vi "Tri-Tri minimum separation.vi"(2 "Triangle 2":T1, 3 "Triangle 1":T1) -> (0 "Minimum separation distance":sgl, 1 "Minimum separation vector\nfrom triangle 2 to triange 1":sgl[](array[numeric]))   [LabVIEW 2014]
uses:
  Typedefs/Triangle.ctl
panel:
  # "PN 13/01/2015"
  # "Vertices"
  # "Edges"
  # "Unit normal"
  # "Edge unit normals"
  # "Vertices"
  # "Edges"
  # "Unit normal"
  # "Edge unit normals"
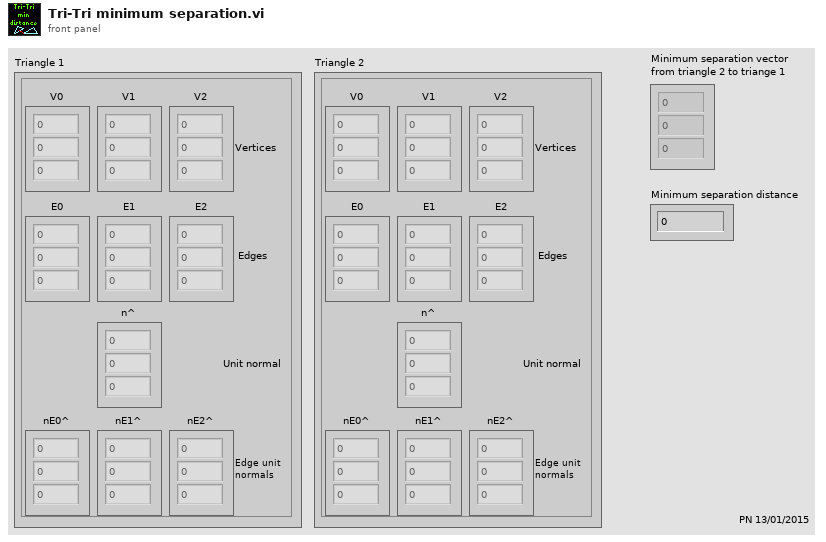
[diagram p1: front panel]
types:
  T1 = typedef "Triangle.ctl" = cluster{"V0":sgl[], "V1":sgl[], "V2":sgl[], "E0":sgl[], "E1":sgl[], "E2":sgl[], "n^":sgl[], "nE0^":sgl[], "nE1^":sgl[], "nE2^":sgl[]}
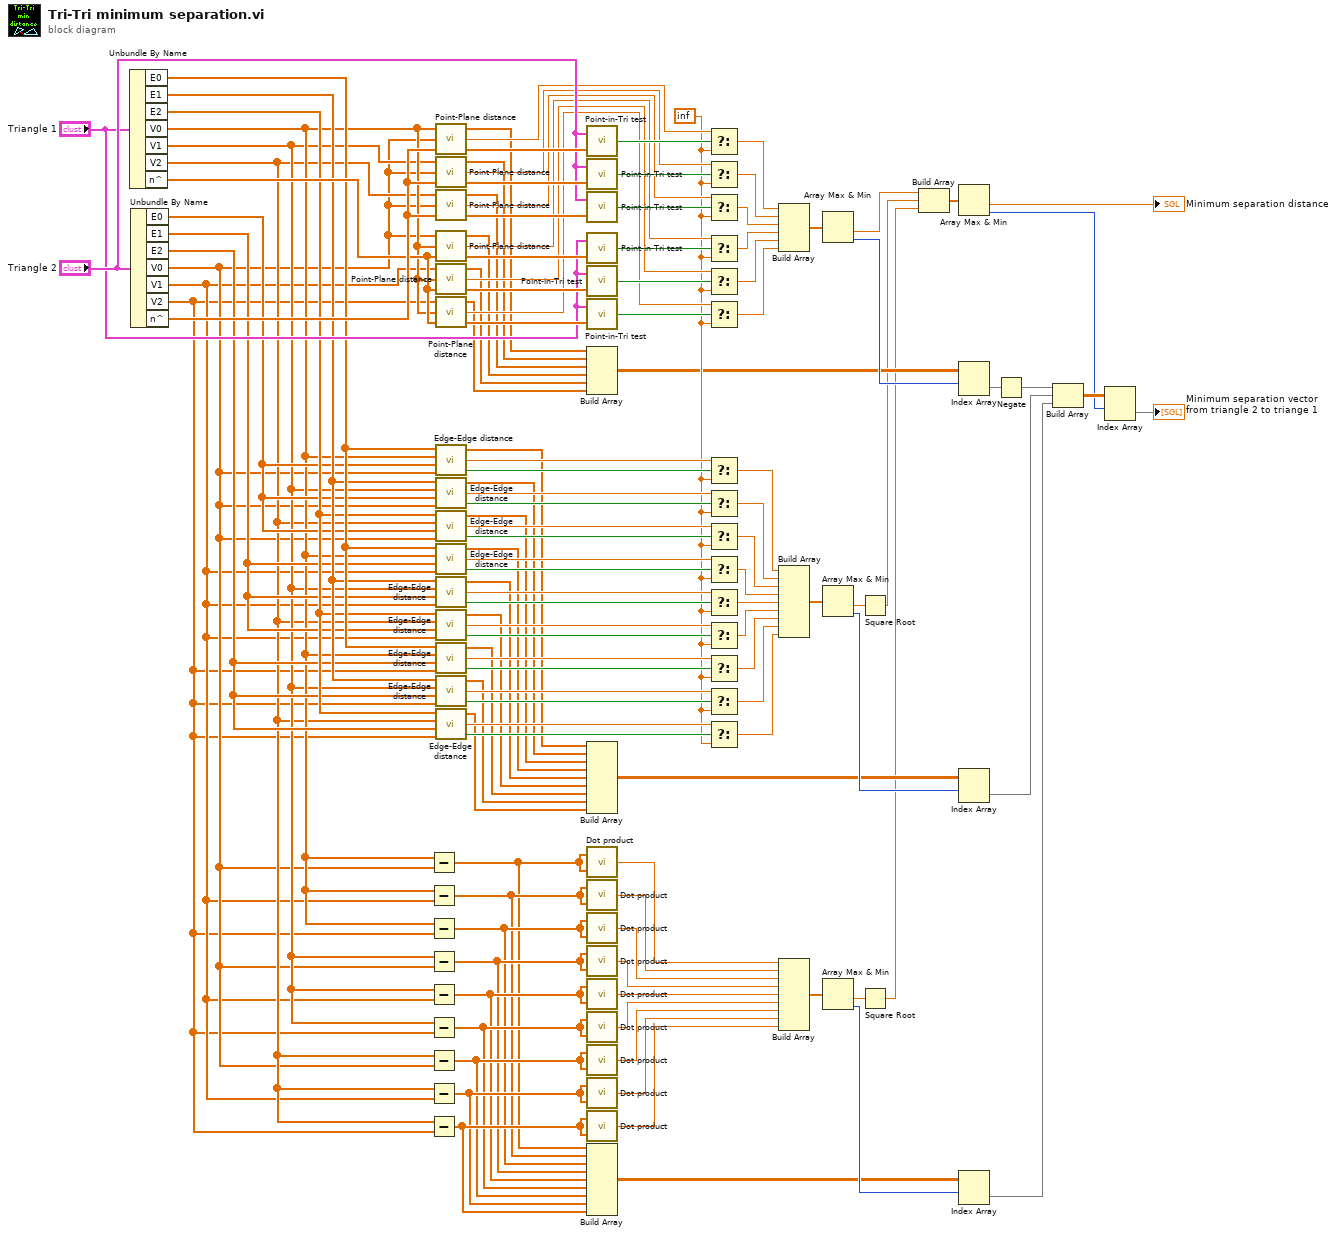
[diagram p0: block diagram]
diagram:
  w78 = sgl inf
  n1 = Unbundle By Name("Triangle 1") -> ("E0"=w114:sgl[], "E1"=w113:sgl[], "E2"=w112:sgl[], "V0"=w77:sgl[], "V1"=w76:sgl[], "V2"=w75:sgl[], "n^"=w115:sgl[])
  n2 = Unbundle By Name("Triangle 2") -> ("E0"=w111:sgl[], "E1"=w110:sgl[], "E2"=w109:sgl[], "V0"=w74:sgl[], "V1"=w73:sgl[], "V2"=w72:sgl[], "n^"=w123:sgl[])
  n3 = Subtract(x=w77, y=w74) -> (x-y=w63:sgl[])
  n4 = Subtract(x=w77, y=w73) -> (x-y=w64:sgl[])
  n5 = Subtract(x=w77, y=w72) -> (x-y=w65:sgl[])
  n6 = Subtract(x=w76, y=w74) -> (x-y=w66:sgl[])
  n7 = Subtract(x=w76, y=w73) -> (x-y=w67:sgl[])
  n8 = Subtract(x=w76, y=w72) -> (x-y=w68:sgl[])
  n9 = Subtract(x=w75, y=w74) -> (x-y=w69:sgl[])
  n10 = Subtract(x=w75, y=w73) -> (x-y=w70:sgl[])
  n11 = Subtract(x=w75, y=w72) -> (x-y=w71:sgl[])
  n12 = call "Point-Plane distance.vi"("Plane normal (unit)"=w123, "Point on plane"=w74, "Point"=w77) -> ("Projected point on plane (along normal)"=w124:sgl[], "| Distance |"=w102:sgl, "Distance vector (from plane)"=w48:sgl[])
  n13 = call "Point-Plane distance.vi"("Plane normal (unit)"=w123, "Point on plane"=w74, "Point"=w76) -> ("Projected point on plane (along normal)"=w122:sgl[], "| Distance |"=w101:sgl, "Distance vector (from plane)"=w49:sgl[])
  n14 = call "Point-Plane distance.vi"("Plane normal (unit)"=w123, "Point on plane"=w74, "Point"=w75) -> ("Projected point on plane (along normal)"=w121:sgl[], "| Distance |"=w100:sgl, "Distance vector (from plane)"=w50:sgl[])
  n15 = call "Point-Plane distance.vi"("Plane normal (unit)"=w115, "Point on plane"=w77, "Point"=w74) -> ("Projected point on plane (along normal)"=w117:sgl[], "| Distance |"=w99:sgl, "Distance vector (from plane)"=w51:sgl[])
  n16 = call "Point-Plane distance.vi"("Plane normal (unit)"=w115, "Point on plane"=w77, "Point"=w73) -> ("Projected point on plane (along normal)"=w118:sgl[], "| Distance |"=w98:sgl, "Distance vector (from plane)"=w52:sgl[])
  n17 = call "Point-Plane distance.vi"("Plane normal (unit)"=w115, "Point on plane"=w77, "Point"=w72) -> ("Projected point on plane (along normal)"=w119:sgl[], "| Distance |"=w97:sgl, "Distance vector (from plane)"=w53:sgl[])
  n18 = call "Edge-Edge distance.vi"("Edge 2 start point"=w74, "Edge 2 (not unit)"=w111, "Edge 1 start point"=w77, "Edge 1 (not unit)"=w114) -> ("Include"=w96:bool, "Distance^2"=w90:sgl, "Distance vector"=w54:sgl[])
  n19 = call "Edge-Edge distance.vi"("Edge 2 start point"=w74, "Edge 2 (not unit)"=w111, "Edge 1 start point"=w76, "Edge 1 (not unit)"=w113) -> ("Include"=w95:bool, "Distance^2"=w89:sgl, "Distance vector"=w55:sgl[])
  n20 = call "Edge-Edge distance.vi"("Edge 2 start point"=w74, "Edge 2 (not unit)"=w111, "Edge 1 start point"=w75, "Edge 1 (not unit)"=w112) -> ("Include"=w94:bool, "Distance^2"=w88:sgl, "Distance vector"=w56:sgl[])
  n21 = call "Edge-Edge distance.vi"("Edge 2 start point"=w73, "Edge 2 (not unit)"=w110, "Edge 1 start point"=w77, "Edge 1 (not unit)"=w114) -> ("Include"=w93:bool, "Distance^2"=w87:sgl, "Distance vector"=w57:sgl[])
  n22 = call "Edge-Edge distance.vi"("Edge 2 start point"=w73, "Edge 2 (not unit)"=w110, "Edge 1 start point"=w76, "Edge 1 (not unit)"=w113) -> ("Include"=w92:bool, "Distance^2"=w86:sgl, "Distance vector"=w58:sgl[])
  n23 = call "Edge-Edge distance.vi"("Edge 2 start point"=w73, "Edge 2 (not unit)"=w110, "Edge 1 start point"=w75, "Edge 1 (not unit)"=w112) -> ("Include"=w91:bool, "Distance^2"=w85:sgl, "Distance vector"=w59:sgl[])
  n24 = call "Edge-Edge distance.vi"("Edge 2 start point"=w72, "Edge 2 (not unit)"=w109, "Edge 1 start point"=w77, "Edge 1 (not unit)"=w114) -> ("Include"=w84:bool, "Distance^2"=w81:sgl, "Distance vector"=w60:sgl[])
  n25 = call "Edge-Edge distance.vi"("Edge 2 start point"=w72, "Edge 2 (not unit)"=w109, "Edge 1 start point"=w76, "Edge 1 (not unit)"=w113) -> ("Include"=w83:bool, "Distance^2"=w80:sgl, "Distance vector"=w61:sgl[])
  n26 = call "Edge-Edge distance.vi"("Edge 2 start point"=w72, "Edge 2 (not unit)"=w109, "Edge 1 start point"=w75, "Edge 1 (not unit)"=w112) -> ("Include"=w82:bool, "Distance^2"=w79:sgl, "Distance vector"=w62:sgl[])
  n27 = call "Point-in-Tri test.vi"("Point"=w124, "Triangle"="Triangle 2") -> ("Point is inside triangle"=w108:bool)
  n28 = call "Point-in-Tri test.vi"("Point"=w122, "Triangle"="Triangle 2") -> ("Point is inside triangle"=w107:bool)
  n29 = call "Point-in-Tri test.vi"("Point"=w121, "Triangle"="Triangle 2") -> ("Point is inside triangle"=w106:bool)
  n30 = call "Point-in-Tri test.vi"("Point"=w117, "Triangle"="Triangle 1") -> ("Point is inside triangle"=w105:bool)
  n31 = call "Point-in-Tri test.vi"("Point"=w118, "Triangle"="Triangle 1") -> ("Point is inside triangle"=w104:bool)
  n32 = call "Point-in-Tri test.vi"("Point"=w119, "Triangle"="Triangle 1") -> ("Point is inside triangle"=w103:bool)
  n33 = Build Array(w48, w49, w50, w51, w52, w53) -> (w15:sgl[][])
  n34 = Build Array(w54, w55, w56, w57, w58, w59, w60, w61, w62) -> (w21:sgl[][])
  n35 = call "Dot product.vi"("B"=w63, "A"=w63) -> ("A . B"=w32:sgl)
  n36 = call "Dot product.vi"("B"=w64, "A"=w64) -> ("A . B"=w31:sgl)
  n37 = call "Dot product.vi"("B"=w65, "A"=w65) -> ("A . B"=w30:sgl)
  n38 = call "Dot product.vi"("B"=w66, "A"=w66) -> ("A . B"=w29:sgl)
  n39 = call "Dot product.vi"("B"=w67, "A"=w67) -> ("A . B"=w28:sgl)
  n40 = call "Dot product.vi"("B"=w68, "A"=w68) -> ("A . B"=w27:sgl)
  n41 = call "Dot product.vi"("B"=w69, "A"=w69) -> ("A . B"=w24:sgl)
  n42 = call "Dot product.vi"("B"=w70, "A"=w70) -> ("A . B"=w25:sgl)
  n43 = call "Dot product.vi"("B"=w71, "A"=w71) -> ("A . B"=w26:sgl)
  n44 = Build Array(w63, w64, w65, w66, w67, w68, w69, w70, w71) -> (w18:sgl[][])
  n45 = Select(t=w102, s=w108, f=w78) -> (s? t:f=w47:sgl)
  n46 = Select(t=w101, s=w107, f=w78) -> (s? t:f=w46:sgl)
  n47 = Select(t=w100, s=w106, f=w78) -> (s? t:f=w45:sgl)
  n48 = Select(t=w99, s=w105, f=w78) -> (s? t:f=w44:sgl)
  n49 = Select(t=w98, s=w104, f=w78) -> (s? t:f=w43:sgl)
  n50 = Select(t=w97, s=w103, f=w78) -> (s? t:f=w42:sgl)
  n51 = Select(t=w90, s=w96, f=w78) -> (s? t:f=w41:sgl)
  n52 = Select(t=w89, s=w95, f=w78) -> (s? t:f=w40:sgl)
  n53 = Select(t=w88, s=w94, f=w78) -> (s? t:f=w39:sgl)
  n54 = Select(t=w87, s=w93, f=w78) -> (s? t:f=w38:sgl)
  n55 = Select(t=w86, s=w92, f=w78) -> (s? t:f=w37:sgl)
  n56 = Select(t=w85, s=w91, f=w78) -> (s? t:f=w36:sgl)
  n57 = Select(t=w81, s=w84, f=w78) -> (s? t:f=w35:sgl)
  n58 = Select(t=w80, s=w83, f=w78) -> (s? t:f=w34:sgl)
  n59 = Select(t=w79, s=w82, f=w78) -> (s? t:f=w33:sgl)
  n60 = Build Array(w47, w46, w45, w44, w43, w42) -> (w16:sgl[])
  n61 = Build Array(w41, w40, w39, w38, w37, w36, w35, w34, w33) -> (w23:sgl[])
  n62 = Build Array(w32, w31, w30, w29, w28, w27, w24, w25, w26) -> (w20:sgl[])
  n63 = Array Max & Min(array=w16) -> (min value=w14:sgl, min index (indices)=w17:i32)  [unwired: 2 out]
  n64 = Array Max & Min(array=w23) -> (min value=w5:sgl, min index (indices)=w22:i32)  [unwired: 2 out]
  n65 = Array Max & Min(array=w20) -> (min value=w3:sgl, min index (indices)=w19:i32)  [unwired: 2 out]
  n66 = Square Root(x=w5) -> (sqrt(x)=w4:sgl)
  n67 = Square Root(x=w3) -> (sqrt(x)=w2:sgl)
  n68 = Build Array(w14, w4, w2) -> (w10:sgl[])
  n69 = Array Max & Min(array=w10) -> (min value=→"Minimum separation distance":sgl, min index (indices)=w8:i32)  [unwired: 2 out]
  n70 = Index Array(array=w15, index (row)=w17) -> (element=w11:sgl[])  [unwired: 1 in]
  n71 = Index Array(array=w21, index (row)=w22) -> (element=w13:sgl[])  [unwired: 1 in]
  n72 = Index Array(array=w18, index (row)=w19) -> (element=w12:sgl[])  [unwired: 1 in]
  n73 = Negate(x=w11) -> (-x=w1:sgl[])
  n74 = Build Array(w1, w13, w12) -> (w9:sgl[][])
  n75 = Index Array(array=w9, index (row)=w8) -> (element=→"Minimum separation vector\nfrom triangle 2 to triange 1":sgl[])  [unwired: 1 in]
